vi "FetchSeries.vi"(8 "error in (no error)":errorcluster, 10 "SeriesRootPath":path=path "C:/data/comics/series", 11 "SeriesURL":string) -> (0 "error out":errorcluster, 3 "Series":T1)   [LabVIEW 2022 SP3]
uses:
  TypeDefs/Series.ctl
  TypeDefs/LoCG_RootURL.ctl
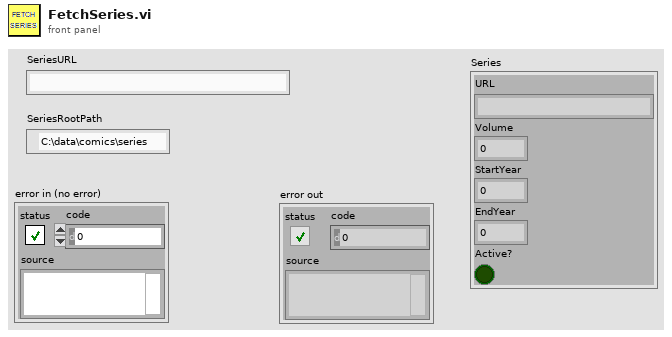
[diagram p1: front panel]
types:
  T1 = typedef "Series.ctl" = cluster{"URL":string, "Volume":i32, "StartYear":i32, "EndYear":i32, "Active?":bool}
  T2 = typedef "LoCG_RootURL.ctl" = string
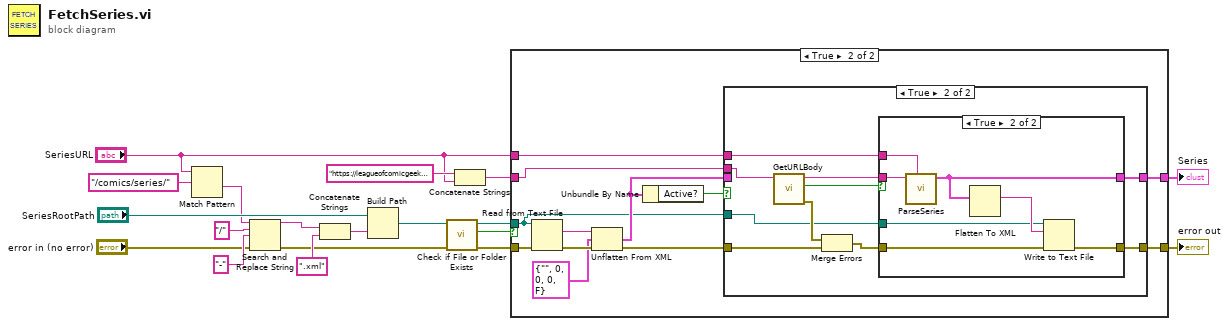
[diagram p0: block diagram]
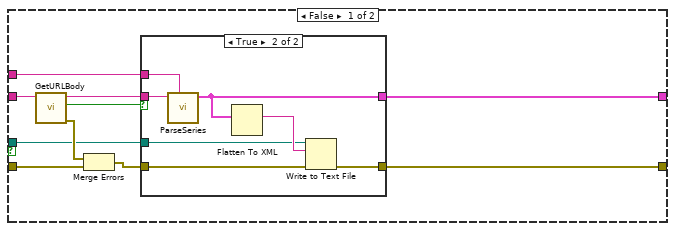
[diagram p2: hidden frame]
diagram:
  n1 = Match Pattern(string="SeriesURL", regular expression="/comics/series/") -> (after substring=w6:string)  [unwired: 1 in, 3 out]
  n2 = Search and Replace String(input string=w6, search string="/", replace string="-" ("replace string (\"\")"), error in="error in (no error)") -> (result string=w3:string, error out=w1:errorcluster)  [unwired: 4 in, 2 out]
  n3 = Concatenate Strings(w3, ".xml" ("string")) -> (w16:string)
  n4 = Build Path(base path="SeriesRootPath", name or relative path=w16) -> (appended path=w14:path)
  n5 = call <vilib>:"Check if File or Folder Exists.vi"("error in (no error)"=w1, "path"=w14) -> ("error out"=w11:errorcluster, "file or folder exists?"=w13:bool, "dup path"=w12:path)  [unwired: 7 in]
  n6 = Concatenate Strings(T2 "https://leagueofcomicgeeks.com/" ("LoCG Root Path"), "SeriesURL") -> (w10:string)
  n7 = case shown="True" w13 {
    tunnel: w12 -> [w20 w40]
    tunnel: w11 -> [w27 w46]
    tunnel: w10 -> [w29 w41]
    tunnel: "SeriesURL" -> [w25 w42]
    tunnel: [w22 w38] -> w8
    tunnel: [w23 w43] -> w7
    frame False {
      n8 = call "GetURLBody.vi"("URL"=w29) -> ("error out"=w28:errorcluster, "Success?"=w24:bool, "body"=w26:string)  [unwired: 7 in, 1 out]
      n9 = Merge Errors(w28, w27) -> (w21:errorcluster)
      n10 = case shown="True" w24 {
        tunnel: w26 -> [_ w37]
        tunnel: w25 -> [_ w36]
        tunnel: [_ w35] -> w23
        tunnel: [w30 w33] -> w22
        tunnel: w21 -> [w30 w32]
        tunnel: w20 -> [_ w31]
        frame False {
        }
        frame True {
          n11 = call "ParseSeries.vi"("Series URl"=w36, "SeriesHTMLBody"=w37) -> ("Series"=w35:T1)  [unwired: 9 in]
          n12 = Flatten To XML(6:w35) -> (2:w34:string)
          n13 = Write to Text File(file (use dialog)=w31, text=w34, error in=w32) -> (error out=w33:errorcluster)  [unwired: 1 in, 2 out]
        }
      }
    }
    frame True {
      n14 = Read from Text File(file (use dialog)=w40, error in=w46) -> (text=w47:string, error out=w49:errorcluster)  [unwired: 2 in, 2 out]
      n15 = Unflatten From XML(xml string=w47, type=T1 {"URL"="", "Volume"=0, "StartYear"=0, "EndYear"=0, "Active?"=FALSE} ("Series"), error in (no error)=w49) -> (value=w44:T1, error out=w39:errorcluster)
      n16 = Unbundle By Name(w44) -> ("Active?"=w45:bool)
      n17 = case shown="True" w45 {
        tunnel: w44 -> [w51 _]
        tunnel: [w51 w52] -> w43
        tunnel: w42 -> [_ w57]
        tunnel: w41 -> [_ w56]
        tunnel: w40 -> [_ w55]
        tunnel: w39 -> [w50 w54]
        tunnel: [w50 w53] -> w38
        frame False {
        }
        frame True {
          n18 = call "GetURLBody.vi"("URL"=w56) -> ("error out"=w61:errorcluster, "Success?"=w59:bool, "body"=w60:string)  [unwired: 7 in, 1 out]
          n19 = Merge Errors(w61, w54) -> (w58:errorcluster)
          n20 = case shown="True" w59 {
            tunnel: w60 -> [_ w69]
            tunnel: w57 -> [_ w68]
            tunnel: [_ w67] -> w52
            tunnel: [w62 w65] -> w53
            tunnel: w58 -> [w62 w64]
            tunnel: w55 -> [_ w63]
            frame False {
            }
            frame True {
              n21 = call "ParseSeries.vi"("Series URl"=w68, "SeriesHTMLBody"=w69) -> ("Series"=w67:T1)  [unwired: 9 in]
              n22 = Flatten To XML(6:w67) -> (2:w66:string)
              n23 = Write to Text File(file (use dialog)=w63, text=w66, error in=w64) -> (error out=w65:errorcluster)  [unwired: 1 in, 2 out]
            }
          }
        }
      }
    }
  }
  "error out" <- w8
  "Series" <- w7
